vi "Read Group Properties.vi"(8 "error in (no error)":errorcluster, 10 "Group Name":string, 11 "TDMS in":refnum<class "TDMS.lvclass">) -> (0 "error out":errorcluster, 3 "TDMS out":refnum<class "TDMS.lvclass">)   [LabVIEW 2019, in "TDMS.lvlib" / "TDMS.lvclass"]
uses:
  TDMS.lvclass
  C:/Users/Public/Documents/Development/builds/Tools/Report.lvlibp/Report.lvclass
  TDMS.lvclass/TDMS.ctl
  builds/Tools/Report.lvlibp/Accessors/Write Report Path.vi
panel:
  out "property values":variant[](array[variant])
  in  "Report Path":path
  out "Property Values":string[](array[string])
  out "property names":string[](array[string])
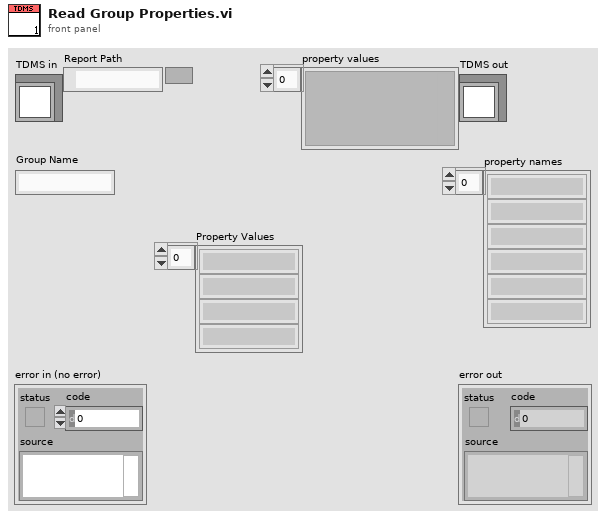
[diagram p1: front panel]
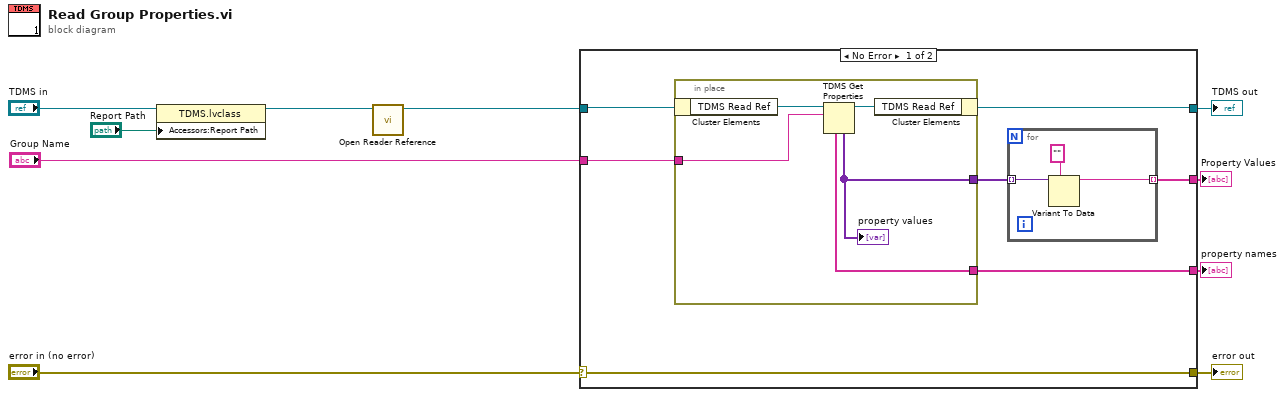
[diagram p0: block diagram]
diagram:
  n1 = property class="TDMS.lvclass"(reference="TDMS in", "Accessors:Report Path"="Report Path") -> (reference out=w2:refnum<class "TDMS.lvclass">)  [unwired: 1 in, 1 out]
  n2 = call "Open Reader Reference.vi"("TDMS in"=w2) -> ("TDMS out"=w3:refnum<class "TDMS.lvclass">)  [unwired: 9 in, 1 out]
  n3 = case shown="No Error" "error in (no error)" {
    selector: "error in (no error)" -> [w17 w27]
    tunnel: [w17 w27] -> w9
    tunnel: [w15 w26] -> w8
    tunnel: w3 -> [w16 w26]
    tunnel: "Group Name" -> [w14 _]
    tunnel: [w13 _] -> w6
    tunnel: [w11 _] -> w5
    frame No Error {
      n4 = in-place {
        in-place-border: w14 -> [w23]
        in-place-border: [w22] -> w13
        in-place-border: [w21] -> w12
        n5 = in-place-cluster #1(w16) -> ("TDMS Read Ref"=w25:refnum<k34>)
        n6 = TDMS Get Properties(10:w23, 11:w25) -> (3:w24:refnum<k34>, 4:w21:variant[], 6:w22:string[])  [unwired: 4 in, 3 out]
        "property values" <- w21
        n7 = in-place-cluster #1("TDMS Read Ref"=w24) -> (w15:refnum<class "TDMS.lvclass">)
      }
      n8 = for {
        tunnel: w12 -> [w20] mode=indexing
        tunnel: [w18] -> w11 mode=indexing
        n9 = Variant To Data(type="", Variant=w20) -> (data=w18:string)  [unwired: 1 in, 1 out]
      }
    }
    frame Error {
    }
  }
  "error out" <- w9
  "TDMS out" <- w8
  "property names" <- w6
  "Property Values" <- w5
